vi "Defined Passed To State.vi"(1 "Defined":bool, 2 "Passed":bool) -> (0 "State":T1)   [LabVIEW 2020, in "Caraya.lvlib" / "Basic Test Manager.lvclass"]
uses:
  Basic Test Manager.lvclass
  Test State.ctl
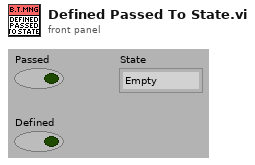
[diagram p1: front panel]
types:
  T1 = typedef "Caraya.lvlib/Basic Test Manager.lvclass/Test State.ctl" = enum16{"Empty", "Unknown", "Fail", "Pass", "Skip", "Error"}
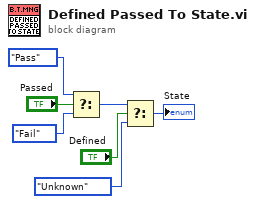
[diagram p0: block diagram]
diagram:
  n1 = Select(t=Test_State."Pass" ("Enum"), s="Passed", f=Test_State."Fail" ("Enum")) -> (s? t:f=w5:T1)
  n2 = Select(t=w5, s="Defined", f=Test_State."Unknown" ("Enum")) -> (s? t:f=→"State":T1)
